vi "Do.vi"(8 "error in (no error)":errorcluster, 10 "Actor in":refnum<class "Actor.lvclass">, 11 "Set Length Msg":refnum<class "Set Length Msg.lvclass">) -> (0 "error out":errorcluster, 2 "Actor out":refnum<class "Actor.lvclass">)   [LabVIEW 2020, in "BNT_DAQmx.lvlib" / "Set Length Msg.lvclass"]
doc: "This VI delivers the message to the actor by calling the appropriate method(s) on the actor."
uses:
  Set Length Msg.lvclass
  <vilib>/ActorFramework/Actor/Actor.lvclass
  C:/Users/holge/Documents/LVP/BNT/PGC/Packages/CSPP_Core/Messages/CSPP_PVUpdate Msg/CSPP_PVUpdate Msg.lvclass
  BNT_DAQmx-MCSV-DOPWM/BNT_DAQmx-MCSV-DOPWM.lvclass
  C:/Program Files (x86)/National Instruments/LabVIEW 2020/vi.lib/ActorFramework/Actor/Actor.lvclass
  CSPP_Core/Messages/CSPP_PVUpdate Msg/CSPP_PVUpdate Msg.lvclass/CSPP_PVUpdate Msg.ctl
  CSPP_Core/Classes/CSPP_ProcessVariables/ProcessVariable/PV.lvclass/PV.ctl
  Set Length Msg.lvclass/Set Length Msg.ctl
  CSPP_Core/Classes/CSPP_ProcessVariables/ProcessVariable/PV.lvclass
  <vilib>/regexp/Match Regular Expression.xnode
  CSPP_Core/Messages/CSPP_PVUpdate Msg/CSPP_PVUpdate Msg.lvclass
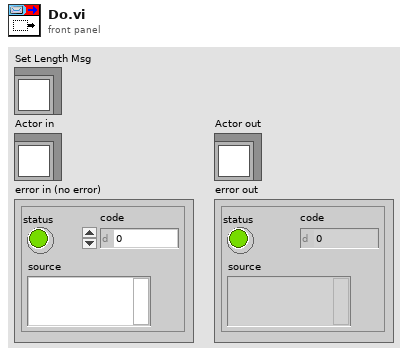
[diagram p1: front panel]
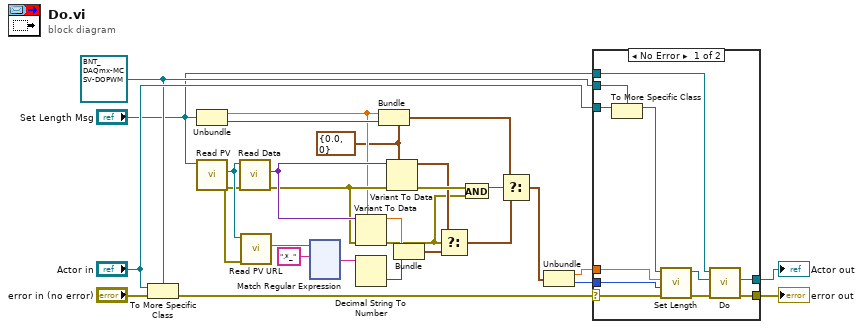
[diagram p0: block diagram]
diagram:
  w1 = cluster{"PWM Length":dbl[unit], "Line":i32} {"PWM Length"=0.0, "Line"=0} ("cluster")
  w25 = refnum<class "BNT_DAQmx-MCSV-DOPWM.lvclass"> refnum ("Actor in")
  n1 = To More Specific Class(target class=w25, reference="Actor in", error in="error in (no error)") -> (error out=w24:errorcluster)  [unwired: 1 out]
  n2 = Unbundle ("Pre-Unbundler")("Set Length Msg") -> (w9:dbl[unit], w19:i32)
  n3 = call "Read PV.vi"("CS++PVUpdate Msg in"="Set Length Msg") -> ("error out"=w12:errorcluster, "PV"=w13:refnum<class "PV.lvclass">)  [unwired: 8 in, 1 out]
  n4 = call "Read Data.vi"("error in (no error)"=w12, "PV in"=w13) -> ("error out"=w10:errorcluster, "Data"=w11:variant)  [unwired: 7 in, 1 out]
  n5 = call "Read PV URL.vi"("error in (no error)"=w12, "PV in"=w13) -> ("PV URL"=w18:string)  [unwired: 7 in, 2 out]
  n6 = xnode "Match Regular Expression"("input string"=w18, "regular expression"=".*_") -> ("after match"=w16:string)  [unwired: 4 in, 4 out]
  n7 = Variant To Data(error in=w10, type=w9, Variant=w11) -> (data=w8:dbl[unit], error out=w4:errorcluster)
  n8 = Decimal String To Number(string=w16) -> (number=w15:i32)  [unwired: 2 in, 1 out]
  n9 = Bundle ("Pre-Bundler")(cluster=w1, "PWM Length"=w9, "Line"=w19) -> (w20:cluster{"PWM Length":dbl[unit], "Line":i32})
  n10 = Variant To Data(error in=w10, type=w1, Variant=w11) -> (data=w7:cluster{"PWM Length":dbl[unit], "Line":i32}, error out=w21:errorcluster)
  n11 = Bundle ("Pre-Bundler")("PWM Length"=w8, w15) -> (w14:cluster{"PWM Length":dbl[unit], i32})  [unwired: 1 in]
  n12 = Select ("MainSelect")(t=w7, s=w4, f=w14) -> (s? t:f=w6:cluster{"PWM Length":dbl[unit], "Line":i32})
  n13 = And(x=w21, y=w4) -> (x .and. y?=w5:bool)
  n14 = Select ("MainSelect")(t=w20, s=w5, f=w6) -> (s? t:f=w3:cluster{"PWM Length":dbl[unit], "Line":i32})
  n15 = Unbundle ("Main-Unbundler")(w3) -> ("PWM Length"=w23:dbl[unit], "Line"=w22:i32)
  n16 = case shown="No Error" w24 {
    selector: w24 -> [w40 w42]
    tunnel: [w35 w42] -> w28
    tunnel: [w36 w41] -> w27
    tunnel: "Actor in" -> [w39 w41]
    tunnel: w25 -> [w38 _]
    tunnel: "Set Length Msg" -> [w32 _]
    tunnel: w23 -> [w31 _]
    tunnel: w22 -> [w30 _]
    frame No Error {
      n17 = To More Specific Class ("To More Specific Class (internal)")(target class=w38, reference=w39) -> (specific class reference=w37:refnum<class "BNT_DAQmx-MCSV-DOPWM.lvclass">)  [unwired: 1 in, 1 out]
      n18 = call "Set Length.vi"("error in"=w40, "Line"=w30, "PWM Length"=w31, "BNT_DAQmx-MCSV-DOPWM in"=w37) -> ("error out"=w34:errorcluster, "BNT_DAQmx-MCSV-DOPWM out"=w33:refnum<class "BNT_DAQmx-MCSV-DOPWM.lvclass">)  [unwired: 6 in]
      n19 = call-parent "Do.vi"("error in (no error)"=w34, "Actor in"=w33, "CS++PVUpdate Msg"=w32) -> ("error out"=w35:errorcluster, "Actor out"=w36:refnum<class "Actor.lvclass">)  [unwired: 7 in]
    }
    frame Error {
    }
  }
  "error out" <- w28
  "Actor out" <- w27
